vi "update.vi"(8 "error in (no error)":errorcluster, 11 "Online_TRAC in":refnum<class "Online_TRAC.lvclass">) -> (0 "error out":errorcluster, 3 "Online_TRAC out":refnum<class "Online_TRAC.lvclass">)   [LabVIEW 2021]
uses:
  Online_TRAC.lvclass
  Online_TRAC.lvclass/Online_TRAC.ctl
  Read Square Cross Sum.vi
  Read Square Esitmated Sum.vi
  Read Square True Sum.vi
  Read N.vi
  Write Square Cross Sum.vi
  Write Square Esitmated Sum.vi
  Write Square True Sum.vi
  Write TRAC.vi
panel:
  in  "Estimate":dbl format="%#_13g"
  in  "True":dbl format="%#_13g"
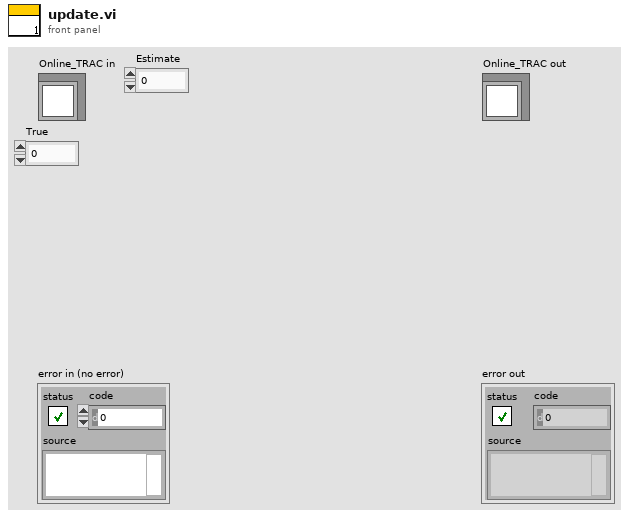
[diagram p1: front panel]
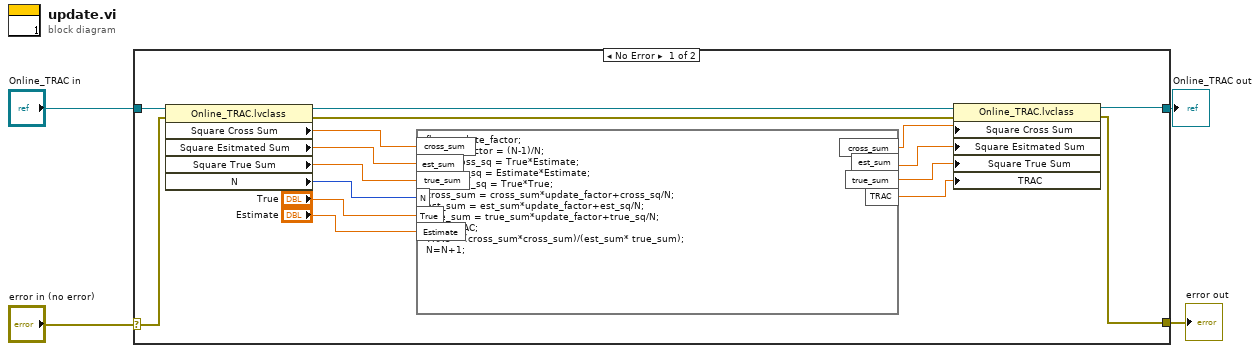
[diagram p0: block diagram]
diagram:
  n1 = case shown="No Error" "error in (no error)" {
    selector: "error in (no error)" -> [w6 w22]
    tunnel: [w5 w22] -> w3
    tunnel: [w8 w21] -> w1
    tunnel: "Online_TRAC in" -> [w20 w21]
    frame No Error {
      n2 = property class="Online_TRAC.lvclass"(reference=w20, error in=w6) -> (reference out=w9:refnum<class "Online_TRAC.lvclass">, error out=w7:errorcluster, "Square Cross Sum"=w19:dbl, "Square Esitmated Sum"=w18:dbl, "Square True Sum"=w17:dbl, "N"=w16:u64)
      n3 = formula code="float update_factor;\nupdate_factor = (N-1)/N;\nfloat cross_sq = True*Estimate;\nfloat est_sq = Estimate*Estimate;\nfloat true_sq = True*True;\ncross_sum = cross_sum*update_factor+cross_sq/N;\nest_sum = est_sum*update_factor+est_sq/N;\ntrue_sum = true_sum*update_factor+true_sq/N;\nfloat TRAC;\nTRAC = (cross_sum*cross_sum)/(est_sum* true_sum);\nN=N+1;"("cross_sum"=w19, "est_sum"=w18, "true_sum"=w17, "N"=w16, "True"="True", "Estimate"="Estimate") -> ("TRAC"=w13:dbl, "cross_sum"=w12:dbl, "est_sum"=w11:dbl, "true_sum"=w10:dbl)
      n4 = property class="Online_TRAC.lvclass"(reference=w9, error in=w7, "Square Cross Sum"=w12, "Square Esitmated Sum"=w11, "Square True Sum"=w10, "TRAC"=w13) -> (reference out=w8:refnum<class "Online_TRAC.lvclass">, error out=w5:errorcluster)
    }
    frame Error {
    }
  }
  "error out" <- w3
  "Online_TRAC out" <- w1
